vi "DIAdem Process Restart Request.vi"(5 "error in (no error)":errorcluster, 7 "DIAdem Queue":T1, 8 "DIAdem Reference":T3) -> (0 "error out":errorcluster, 2 "Script Result":string, 3 "DIAdem Reference":T3)   [LabVIEW 2011]
uses:
  <vilib>/ExportToExcel/DIAdem Reference.ctl
  DIAdem Daemon Queue.ctl
  DIAdem Daemon Script Type.ctl
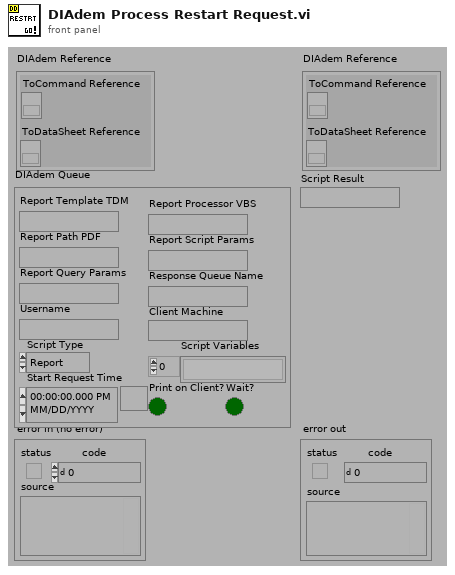
[diagram p1: front panel]
types:
  T1 = typedef "DIAdem Daemon Queue.ctl" = cluster{"Report Template TDM":path, "Report Processor VBS":path, "Report Path PDF":path, "Report Script Params":string, "Username":string, "Script Type":T2, "Report Query Params":string, "Client Machine":string, "Print on Client?":bool, "Response Queue Name":string, "Script Variables":string[], "Start Request Time":timestamp, "Wait?":bool}
  T2 = typedef "DIAdem Daemon Script Type.ctl" = enum16{"Report", "Query", "Script", "Datasheet", "Append", "Restart", "Stop"}
  T3 = typedef "DIAdem Reference.ctl" = cluster{"ToCommand Reference":refnum<k7>, "ToDataSheet Reference":refnum<k7>}
  T4 = cluster{"ToCommand Reference":bool, "ToDataSheet Reference":bool}
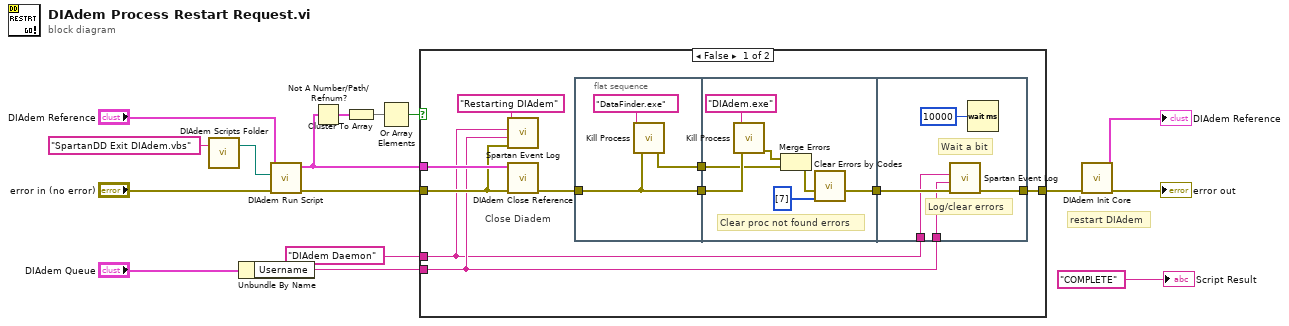
[diagram p0: block diagram]
diagram:
  # "restart DIAdem"
  n1 = call "DIAdem Scripts Folder.vi"("Relative Path (\"\" - Folder)"="SpartanDD Exit DIAdem.vbs" ("Relative Path (\"\" - Folder)")) -> ("Scripts Folder"=w5:path)  [unwired: 2 out]
  n2 = Unbundle By Name("DIAdem Queue") -> ("Username"=w2:string)
  n3 = call "DIAdem Run Script.vi"("error in (no error)"="error in (no error)", "script file"=w5, "DIAdem Reference"="DIAdem Reference") -> ("error out"=w11:errorcluster, "DIAdem Reference"=w10:T3)  [unwired: 7 out]
  n4 = Not A Number/Path/Refnum?(number/path/refnum=w10) -> (NaN/Path/Refnum?=w12:T4)
  n5 = Cluster To Array(cluster=w12) -> (array=w13:bool[])
  n6 = Or Array Elements(Boolean array=w13) -> (logical OR=w14:bool)
  n7 = case shown="False" w14 {
    tunnel: w11 -> [w19 w42]
    tunnel: [w24 w42] -> w9
    tunnel: w10 -> [w26 _]
    tunnel: "DIAdem Daemon" ("name (unnamed)") -> [w17 _]
    tunnel: w2 -> [w18 _]
    frame False {
      # "Close Diadem"
      n8 = call "Spartan Event Log.vi"("error in (no error)"=w19, "username (\"\")"=w18, "module (\"\")"=w17, "message (\"\")"="Restarting DIAdem") -> ()  [unwired: 1 in, 4 out]
      n9 = call <vilib>:"DIAdem Close Reference.vi"("error in (no error)"=w19, "DIAdem Reference"=w26) -> ("error out"=w23:errorcluster)  [unwired: 9 out]
      n10 = flat-sequence {
        tunnel: w23 -> [w29]
        tunnel: [w29] -> w22
        tunnel: [w28] -> w20
        tunnel: w22 -> [w36]
        tunnel: [w31] -> w21
        tunnel: w20 -> [w34]
        tunnel: [w39] -> w24
        tunnel: w21 -> [w40]
        tunnel: w18 -> [w38]
        tunnel: w17 -> [w37]
        frame #0 {
          n11 = call "Kill Process.vi"("error in (no error)"=w29, "Name of Process to kill (\"\")"="DataFinder.exe" ("Name of Process to kill (\"\")")) -> ("error out"=w28:errorcluster)  [unwired: 5 out]
        }
        frame #1 {
          # "Clear proc not found errors"
          n12 = call "Kill Process.vi"("error in (no error)"=w36, "Name of Process to kill (\"\")"="DIAdem.exe" ("Name of Process to kill (\"\")")) -> ("error out"=w35:errorcluster)  [unwired: 5 out]
          n13 = Merge Errors(w35, w34) -> (w32:errorcluster)
          n14 = call "Clear Errors by Codes.vi"("Error Codes\nto Clear (Empty)"=i32[] [7] ("Error Codes\nto Clear (Empty)"), "error in (no error)"=w32) -> ("error out"=w31:errorcluster)  [unwired: 5 out]
        }
        frame #2 {
          # "Log/clear errors"
          # "Wait a bit"
          n15 = call "Spartan Event Log.vi"("error in (no error)"=w40, "username (\"\")"=w38, "module (\"\")"=w37) -> ("error out"=w39:errorcluster)  [unwired: 2 in, 3 out]
          n16 = Wait (ms)(milliseconds to wait=u32 10000) -> ()  [unwired: 1 out]
        }
      }
    }
    frame True {
    }
  }
  n17 = call "DIAdem Init Core.vi"("error in"=w9) -> ("error out"=→"error out":errorcluster, "DIAdem Reference"=→"DIAdem Reference":T3)  [unwired: 9 out]
  "Script Result" <- "COMPLETE" ("Script Result")
